vi "Material_Traceability.vi"() -> ()   [LabVIEW 2020]
doc: "Fonction :\n\nCe modèle peut être intégré très facilement à un subpannel à l'aide des fonctions de la palette Code Template >> Dynamic VI and Subpanel de la VIBOX"
uses:
  System.Windows.Forms
  Program Files (x86)/National Instruments/LabVIEW 2020/examples/DataGrid for LabVIEW/DataGrid.lvlib
panel:
  in  "追溯工位":bool
  in  "追溯总成":bool
  in  "搜索按钮":bool
  in  "追溯码":string
  out "Stop<user event>":refnum<user-event>
  in  "物料":refnum<k24>(container)
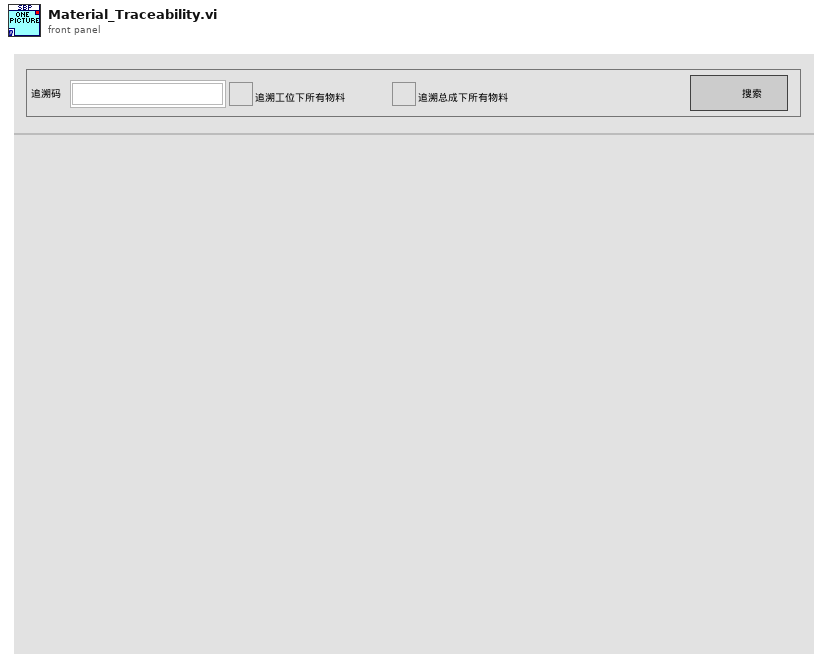
[diagram p1: front panel]
types:
  T1 = typedef "DataGrid.lvlib/GridColumn.lvclass/ColumnDefinition.ctl" = cluster{"name":string, "caption":string, "datatype":T2, "Params":string, "AutoSizeMode":i32, "FillWeight":sgl, "MinWidth":u32, "tooltip":string}
  T2 = typedef "DataGrid.lvlib/GridColumn.lvclass/ColumnType.ctl" = enum16{"string", "image", "check", "numeric", "timestamp", "button", "combo", "link"}
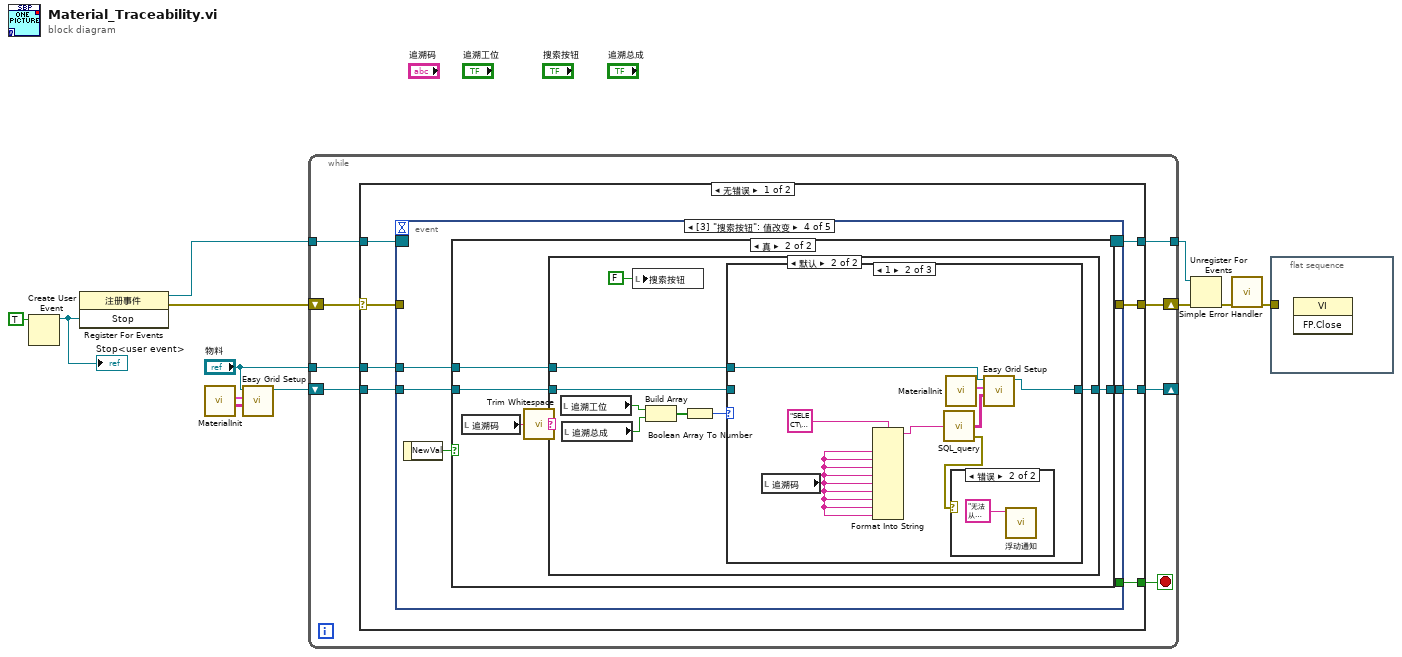
[diagram p0: block diagram]
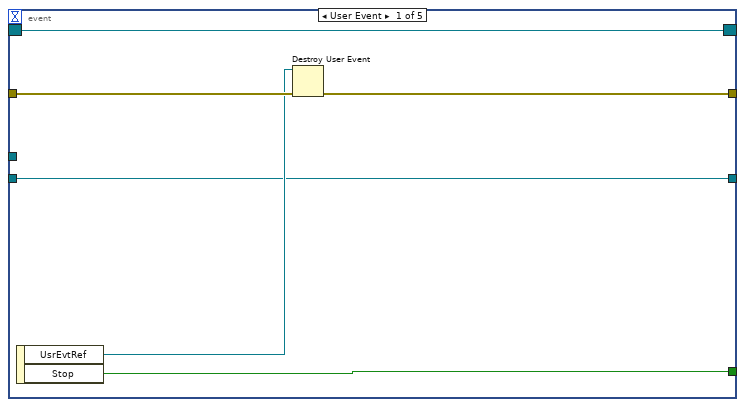
[diagram p2: hidden frame]
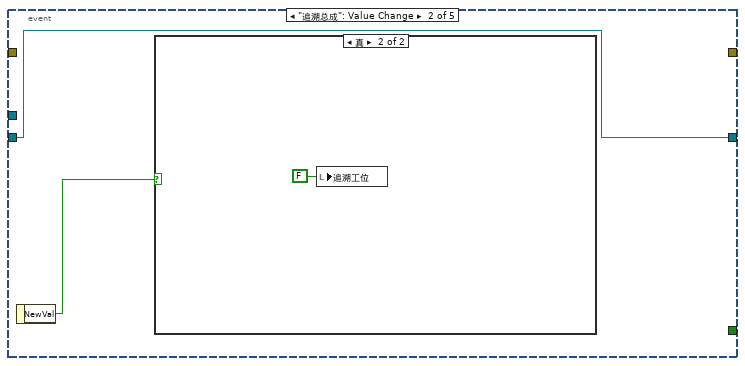
[diagram p3: hidden frame]
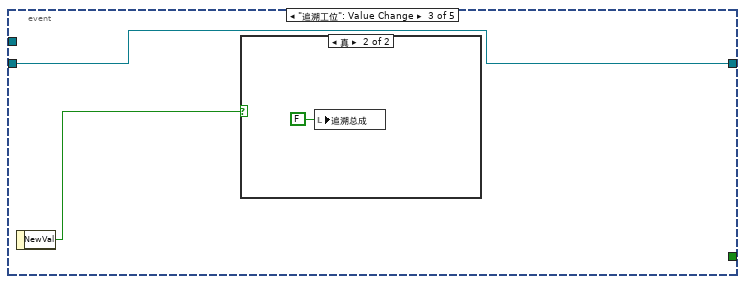
[diagram p5: hidden frame]
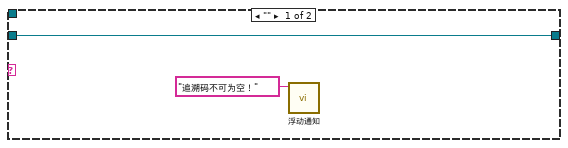
[diagram p8: hidden frame]
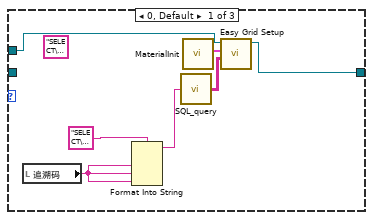
[diagram p9: hidden frame]
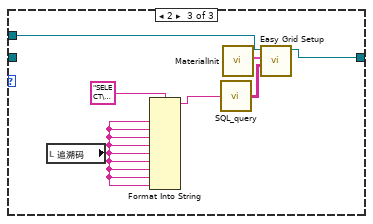
[diagram p11: hidden frame]
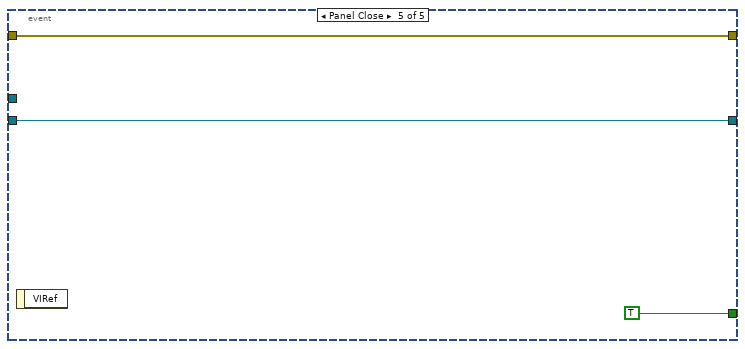
[diagram p12: hidden frame]
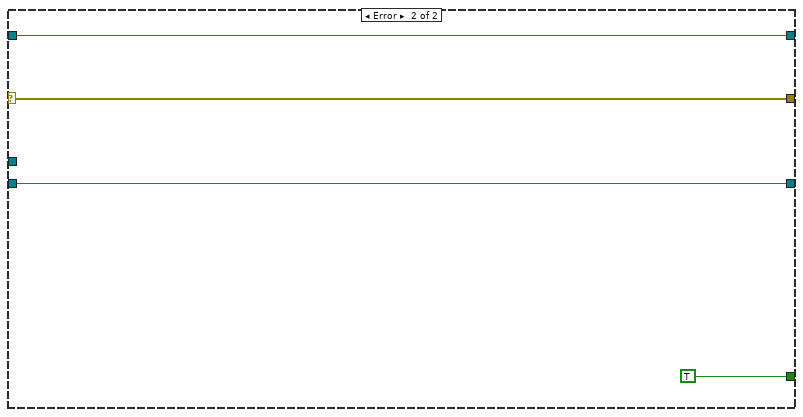
[diagram p13: hidden frame]
diagram:
  n1 = Create User Event(user event datatype=TRUE ("Stop")) -> (user event=w10:refnum<user-event>)  [unwired: 1 in, 1 out]
  "Stop<user event>" <- w10
  n2 = register-events(w10) -> (reference out=w9:refnum<event-registration>, error out=w5:errorcluster)  [unwired: 2 in]
  n3 = call "MaterialInit.vi"() -> ("DataSource Data"=w3:string[][], "ColumnSetup"=w4:T1[])  [unwired: 10 in]
  n4 = call <vilib>:"Easy Grid Setup.vi"("DataSource Data"=w3, "ColumnSetup"=w4, "DataGridView"="物料") -> ("DataGrid out"=w2:refnum<class "DataGridView.lvclass">)  [unwired: 5 in, 3 out]
  n5 = while {
    tunnel: w9 -> [w17]
    tunnel: [w16] -> w12
    shift-right: [w19] -> w8
    shift-left: w5 -> [w20]
    shift-right: [w14] -> _
    shift-left: w2 -> [w15]
    tunnel: "物料" -> [w13]
    stop <- w18 stop-if-true
    n6 = case shown="无错误" w20 {
      selector: w20 -> [w25 w89]
      tunnel: [w24 w89] -> w19
      tunnel: [w26 TRUE] -> w18
      tunnel: w17 -> [w27 w88]
      tunnel: [w28 w88] -> w16
      tunnel: w15 -> [w23 w87]
      tunnel: [w22 w87] -> w14
      tunnel: w13 -> [w21 _]
      frame No Error {
        n7 = event shown="[3] \"搜索按钮\": 值改变" {
          selector: w27 -> [w34 _ _ _ _]
          dyn-events: [w34 _ _ _ _] -> w28
          timeout: _ -> [_ _ _ _ _]
          tunnel: [w31 _ _ _ TRUE ("Stop")] -> w26
          tunnel: w25 -> [w33 _ _ _ w85]
          tunnel: [w30 _ _ _ w85] -> w24
          tunnel: w23 -> [w29 w35 w38 w43 w84]
          tunnel: [w29 w35 w38 w42 w84] -> w22
          tunnel: w21 -> [_ _ _ w41 _]
          event User Event {
            n8 = event-data() -> ("UsrEvtRef"=w32:refnum<user-event>, "Stop"=w31:bool)  [unwired: 1 out]
            n9 = Destroy User Event(user event=w32, error in=w33) -> (error out=w30:errorcluster)
          }
          event "追溯总成": Value Change {
            n10 = event-data() -> ("NewVal"=w36:bool)  [unwired: 1 out]
            n11 = case shown="真" w36 {
              frame False {
              }
              frame True {
                n12 = local write "追溯工位"(FALSE ("追溯工位")) -> ()
              }
            }
          }
          event "追溯工位": Value Change {
            n13 = event-data() -> ("NewVal"=w39:bool)  [unwired: 1 out]
            n14 = case shown="真" w39 {
              frame False {
              }
              frame True {
                n15 = local write "追溯总成"(FALSE ("追溯总成")) -> ()
              }
            }
          }
          event "搜索按钮": Value Change {
            n16 = event-data() -> ("NewVal"=w44:bool)  [unwired: 1 out]
            n17 = case shown="真" w44 {
              tunnel: w43 -> [w45 w48]
              tunnel: [w45 w49] -> w42
              tunnel: w41 -> [_ w50]
              frame False {
              }
              frame True {
                n18 = local read "追溯码"() -> (w47:string)
                n19 = call <vilib>:"Trim Whitespace.vi"("string"=w47) -> ("trimmed string"=w46:string)  [unwired: 1 in]
                n20 = case shown="默认" w46 {
                  tunnel: w50 -> [_ w55]
                  tunnel: [w52 w54] -> w49
                  tunnel: w48 -> [w52 w53]
                  frame "" {
                    n21 = call "浮动通知.vi"("通知内容"="追溯码不可为空！") -> ()  [unwired: 11 in]
                  }
                  frame Default {
                    n22 = local read "追溯工位"() -> (w59:bool)
                    n23 = local read "追溯总成"() -> (w58:bool)
                    n24 = local write "搜索按钮"(FALSE ("搜索按钮")) -> ()
                    n25 = Build Array(w59, w58) -> (w57:bool[])
                    n26 = Boolean Array To Number(Boolean array=w57) -> (number=w56:u32)
                    n27 = case shown="1" w56 {
                      tunnel: w55 -> [w66 w71 w80]
                      tunnel: [w67 w70 w81] -> w54
                      tunnel: w53 -> [_ _ _]
                      frame 0, Default {
                        (unwired) "SELECT\n\tdbo.[物料].[生产编号],\n\tdbo.[物料].[产品型号],\n\tdbo.[物料].[设备型号],\n\tdbo.[物料].[物料名称],\n\tdbo.[物料].[物料追溯码],\n\tdbo.[物料].[工位追溯码],\n\tdbo.[物料].[总成追溯码]\nFROM\ndbo.[物料]\nWHERE\ndbo.[物料].[物料追溯码] like '%%%s%%' OR\ndbo.[物料].[总成追溯码] like '%%%s%%' OR\ndbo.[物料].[工位追溯码] like '%%%s%%'\n"
                        n28 = local read "追溯码"() -> (w63:string)
                        n29 = Format Into String(format string="SELECT\n\tdbo.[物料].[生产编号],\n\tdbo.[物料].[产品型号],\n\tdbo.[物料].[设备型号],\n\tdbo.[物料].[物料名称],\n\tdbo.[物料].[物料追溯码],\n\tdbo.[物料].[工位追溯码],\n\tdbo.[物料].[总成追溯码]\nFROM\ndbo.[物料]\nWHERE\ndbo.[物料].[物料追溯码] like N'%%%s%%' OR\ndbo.[物料].[总成追溯码] like N'%%%s%%' OR\ndbo.[物料].[工位追溯码] like N'%%%s%%'\n", w63, w63, w63) -> (resulting string=w62:string)  [unwired: 2 in, 1 out]
                        n30 = call "SQL_query.vi"("SQL query"=w62) -> ("data"=w64:string[][])  [unwired: 3 in, 1 out]
                        n31 = call "MaterialInit.vi"() -> ("ColumnSetup"=w65:T1[])  [unwired: 10 in, 1 out]
                        n32 = call <vilib>:"Easy Grid Setup.vi"("DataSource Data"=w64, "ColumnSetup"=w65, "DataGridView"=w66) -> ("DataGrid out"=w67:refnum<class "DataGridView.lvclass">)  [unwired: 5 in, 3 out]
                      }
                      frame 1 {
                        n33 = local read "追溯码"() -> (w73:string)
                        n34 = Format Into String(format string="SELECT\n\tdbo.[物料].[生产编号],\n\tdbo.[物料].[产品型号],\n\tdbo.[物料].[设备型号],\n\tdbo.[物料].[物料名称],\n\tdbo.[物料].[物料追溯码],\n\tdbo.[物料].[工位追溯码],\n\tdbo.[物料].[总成追溯码]\nFROM\n\tdbo.[物料]\nWHERE\n\tdbo.[物料].[物料追溯码] = (\n\t\tSELECT DISTINCT\n\t\t\tdbo.[物料].[工位追溯码]\n\t\tFROM\n\t\t\tdbo.[物料]\n\t\tWHERE\n\t\t\tdbo.[物料].[物料追溯码] = N'%s'\n\t\tOR dbo.[物料].[工位追溯码] = N'%s'\n\t\tOR dbo.[物料].[总成追溯码] = N'%s'\n\t)\nOR dbo.[物料].[工位追溯码] = (\n\tSELECT DISTINCT\n\t\tdbo.[物料].[工位追溯码]\n\tFROM\n\t\tdbo.[物料]\n\tWHERE\n\t\tdbo.[物料].[物料追溯码] = N'%s'\n\tOR dbo.[物料].[工位追溯码] = N'%s'\n\tOR dbo.[物料].[总成追溯码] = N'%s'\n)\nOR dbo.[物料].[总成追溯码] = (\n\tSELECT DISTINCT\n\t\tdbo.[物料].[工位追溯码]\n\tFROM\n\t\tdbo.[物料]\n\tWHERE\n\t\tdbo.[物料].[物料追溯码] = N'%s'\n\tOR dbo.[物料].[工位追溯码] = N'%s'\n\tOR dbo.[物料].[总成追溯码] = N'%s'\n)", w73, w73, w73, w73, w73, w73, w73, w73, w73) -> (resulting string=w72:string)  [unwired: 2 in, 1 out]
                        n35 = call "SQL_query.vi"("SQL query"=w72) -> ("error out"=w68:errorcluster, "data"=w74:string[][])  [unwired: 3 in]
                        n36 = call "MaterialInit.vi"() -> ("ColumnSetup"=w75:T1[])  [unwired: 10 in, 1 out]
                        n37 = case shown="错误" w68 {
                          frame No Error {
                          }
                          frame Error {
                            n38 = call "浮动通知.vi"("通知内容"="无法从总成码追溯至工位！") -> ()  [unwired: 11 in]
                          }
                        }
                        n39 = call <vilib>:"Easy Grid Setup.vi"("DataSource Data"=w74, "ColumnSetup"=w75, "DataGridView"=w71) -> ("DataGrid out"=w70:refnum<class "DataGridView.lvclass">)  [unwired: 5 in, 3 out]
                      }
                      frame 2 {
                        n40 = local read "追溯码"() -> (w79:string)
                        n41 = Format Into String(format string="SELECT\n\tdbo.[物料].[生产编号],\n\tdbo.[物料].[产品型号],\n\tdbo.[物料].[设备型号],\n\tdbo.[物料].[物料名称],\n\tdbo.[物料].[物料追溯码],\n\tdbo.[物料].[工位追溯码],\n\tdbo.[物料].[总成追溯码]\nFROM\n\tdbo.[物料]\nWHERE\n\tdbo.[物料].[物料追溯码] = (\n\t\tSELECT DISTINCT\n\t\t\tdbo.[物料].[总成追溯码]\n\t\tFROM\n\t\t\tdbo.[物料]\n\t\tWHERE\n\t\t\tdbo.[物料].[物料追溯码] = N'%s'\n\t\tOR dbo.[物料].[工位追溯码] = N'%s'\n\t\tOR dbo.[物料].[总成追溯码] = N'%s'\n\t)\nOR dbo.[物料].[工位追溯码] = (\n\tSELECT DISTINCT\n\t\tdbo.[物料].[总成追溯码]\n\tFROM\n\t\tdbo.[物料]\n\tWHERE\n\t\tdbo.[物料].[物料追溯码] = N'%s'\n\tOR dbo.[物料].[工位追溯码] = N'%s'\n\tOR dbo.[物料].[总成追溯码] = N'%s'\n)\nOR dbo.[物料].[总成追溯码] = (\n\tSELECT DISTINCT\n\t\tdbo.[物料].[总成追溯码]\n\tFROM\n\t\tdbo.[物料]\n\tWHERE\n\t\tdbo.[物料].[物料追溯码] = N'%s'\n\tOR dbo.[物料].[工位追溯码] = N'%s'\n\tOR dbo.[物料].[总成追溯码] = N'%s'\n)", w79, w79, w79, w79, w79, w79, w79, w79, w79) -> (resulting string=w78:string)  [unwired: 2 in, 1 out]
                        n42 = call "SQL_query.vi"("SQL query"=w78) -> ("data"=w82:string[][])  [unwired: 3 in, 1 out]
                        n43 = call "MaterialInit.vi"() -> ("ColumnSetup"=w83:T1[])  [unwired: 10 in, 1 out]
                        n44 = call <vilib>:"Easy Grid Setup.vi"("DataSource Data"=w82, "ColumnSetup"=w83, "DataGridView"=w80) -> ("DataGrid out"=w81:refnum<class "DataGridView.lvclass">)  [unwired: 5 in, 3 out]
                      }
                    }
                  }
                }
              }
            }
          }
          event Panel Close {
            n45 = event-data() -> ()  [unwired: 2 out]
          }
        }
      }
      frame Error {
      }
    }
  }
  n46 = Unregister For Events(event registration refnum=w12, error in=w8) -> (error out=w11:errorcluster)
  n47 = call <vilib>:"Simple Error Handler.vi"("error in (no error)"=w11) -> ("error out"=w6:errorcluster)  [unwired: 1 in, 7 out]
  n48 = flat-sequence {
    tunnel: w6 -> [_]
    frame #0 {
      n49 = invoke class="VI" method="FP.Close"() -> ()  [unwired: 3 in, 3 out]
    }
  }
